vi "PeriodicFilter-Format Result.vi"(7 "Time Format String":string="%<%Y/%m/%d %H:%M:%S%3u>T", 8 "Filtered":bool, 9 "Additional Info":string[](array[string]), 10 "Current Time":timestamp, 11 "Cross CSM Data In":T1) -> (3 "States":string)   [LabVIEW 2017, in "Communicable State Machine.lvlib"]
uses:
  Communicable State Machine.lvlib
  _Support/Typedef/_CSM_GlobalLog_MSG.ctl
  _Support/Typedef/_CSM_Response Source Message.ctl
  _Support/Typedef/_CSM_GlobalLog_MSG_TYPE.ctl
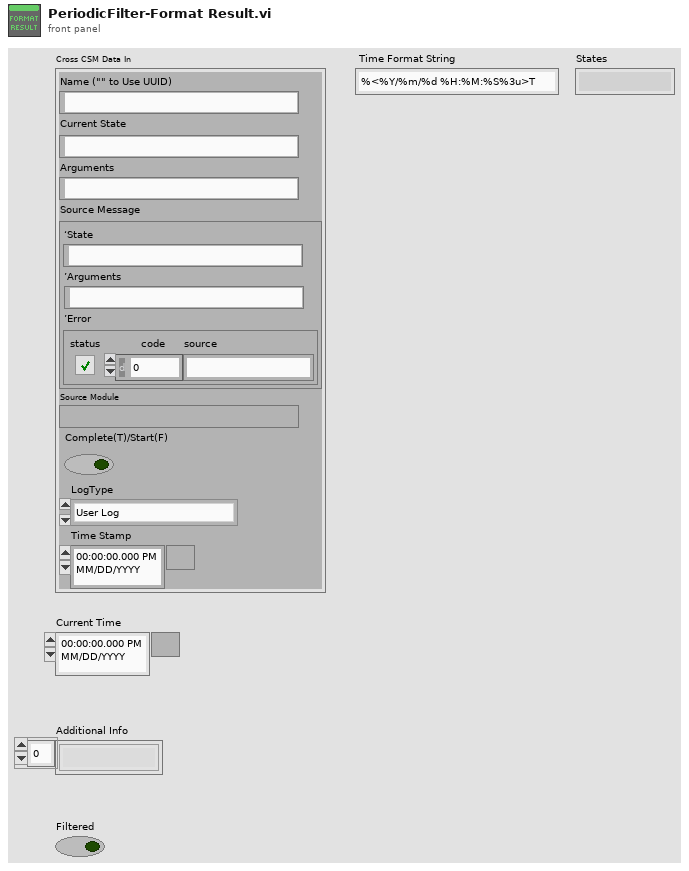
[diagram p1: front panel]
types:
  T1 = typedef "Communicable State Machine.lvlib/_CSM_GlobalLog_MSG.ctl" = cluster{"Name (\"\" to Use UUID)":string, "Current State":string, "Arguments":string, "Source Message":T2, "Source Module":string, "Complete(T)/Start(F)":bool, "LogType":T3, "Time Stamp":timestamp}
  T2 = typedef "Communicable State Machine.lvlib/_CSM_Response Source Message.ctl" = cluster{"‘State":string, "’Arguments":string, "’Error":errorcluster}
  T3 = typedef "Communicable State Machine.lvlib/_CSM_GlobalLog_MSG_TYPE.ctl" = enum16{"User Log", "State Change", "Status", "Interrupt", "Register", "Unregister", "Error Log", "Module Created", "Module Destroyed", "Async Message", "No-Rep Async Message", "Sync Message"}
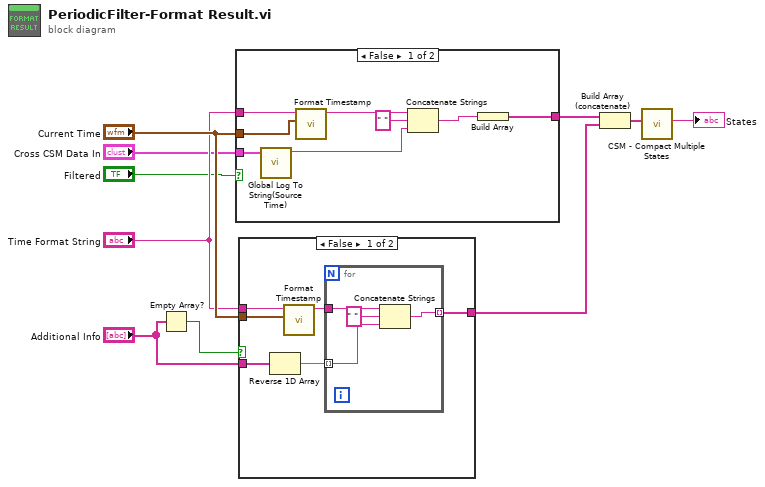
[diagram p0: block diagram]
diagram:
  n1 = Empty Array?(array="Additional Info") -> (empty?=w1:bool)
  n2 = case shown="False" "Filtered" {
    tunnel: "Cross CSM Data In" -> [w18 _]
    tunnel: [w11 _] -> w5
    tunnel: "Time Format String" -> [w15 _]
    tunnel: "Current Time" -> [w14 _]
    frame False {
      n3 = call "Global Log To String(Source Time).vi"("Log"=w18) -> ("Log String"=w13:string)  [unwired: 9 in]
      n4 = call "Format Timestamp.vi"("Timestamp"=w14, "Format String"=w15) -> ("String"=w16:string)  [unwired: 9 in]
      n5 = Concatenate Strings(w16, " " ("string"), w13) -> (w12:string)
      n6 = Build Array(w12) -> (w11:string[])
    }
    frame True {
    }
  }
  n7 = case shown="False" w1 {
    tunnel: "Current Time" -> [w24 _]
    tunnel: "Additional Info" -> [w23 _]
    tunnel: "Time Format String" -> [w22 _]
    tunnel: [w21 _] -> w2
    frame False {
      n8 = Reverse 1D Array(array=w23) -> (reversed array=w19:string[])
      n9 = call "Format Timestamp.vi"("Timestamp"=w24, "Format String"=w22) -> ("String"=w20:string)  [unwired: 9 in]
      n10 = for {
        tunnel: w19 -> [w28] mode=indexing
        tunnel: w20 -> [w26]
        tunnel: [w25] -> w21 mode=indexing
        n11 = Concatenate Strings(w26, " " ("string"), w28) -> (w25:string)
      }
    }
    frame True {
    }
  }
  n12 = Build Array (concatenate)(w5, w2) -> (w3:string[])
  n13 = call "CSM - Compact Multiple States.vi"("Multiple States"=w3) -> ("States"=→"States":string)  [unwired: 9 in]
